vi "Create Music Element.vi"(8 "error in (no error)":errorcluster, 10 "Name":string, 11 "MusicElement in":refnum<class "MusicElement.lvclass">) -> (0 "error out":errorcluster, 3 "MusicElement out":refnum<class "MusicElement.lvclass">)   [LabVIEW 2015, in "MusicElement.lvclass"]
uses:
  MusicElement.lvclass
  MusicElement.lvclass/MusicElement.ctl
  Write Name.vi
  Write UID.vi
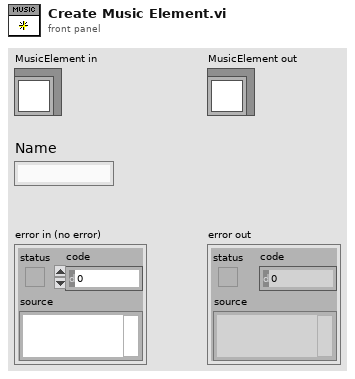
[diagram p1: front panel]
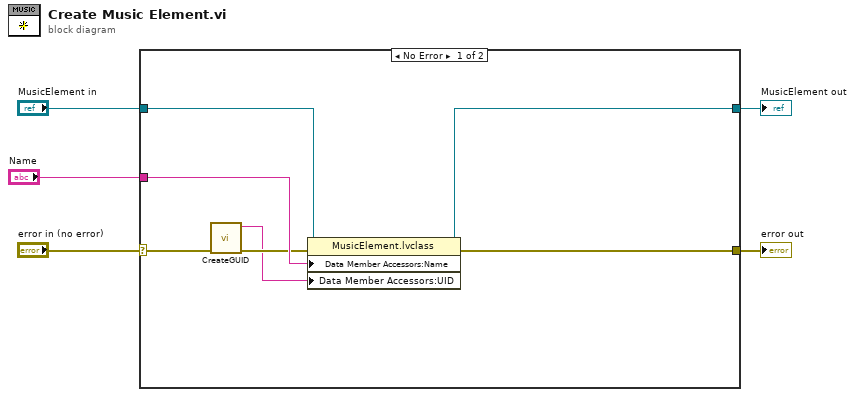
[diagram p0: block diagram]
diagram:
  n1 = case shown="No Error" "error in (no error)" {
    selector: "error in (no error)" -> [w8 w14]
    tunnel: [w9 w14] -> w4
    tunnel: [w11 w13] -> w2
    tunnel: "MusicElement in" -> [w12 w13]
    tunnel: "Name" -> [w10 _]
    frame No Error {
      n2 = call "CreateGUID.vi"("error in (no error)"=w8) -> ("error out"=w7:errorcluster, "GUID"=w6:string)  [unwired: 9 in]
      n3 = property class="MusicElement.lvclass"(reference=w12, error in=w7, "Data Member Accessors:Name"=w10, "Data Member Accessors:UID"=w6) -> (reference out=w11:refnum<class "MusicElement.lvclass">, error out=w9:errorcluster)
    }
    frame Error {
    }
  }
  "error out" <- w4
  "MusicElement out" <- w2
